vi "UPCONVERSION.vi"() -> ()   [LabVIEW 2011]
uses:
  Control 1.ctl
  Control 2.ctl
  <vilib>/Utility/file.llb/Write To Spreadsheet File (DBL).vi
panel:
  out "error out":errorcluster
  out "No of Scan":i32
  in  "Stop Taking Data":bool
  in  "UP CONVERSION":T1(tab)
  in  "Position (mm)":dbl
  out "Current position (mm)":dbl
  in  "Start Data Accusition":bool
  out "Position Time Zero":dbl
  in  "Path for Transients":T2="C:\\Users\\Labuser\\Desktop\\Upconversion_data\\"
  in  "Path for final Averaged Data":T3=path "C:/Users/Labuser/Desktop/Upconversion_data/final"
  in  "50 fs":i32
  in  "250 fs":i32
  in  "1ps":i32
  in  "5ps":i32
  out "GRAPH":T4(graph)
  out "XY Graph":cluster{"Y":dbl[], "Y":dbl[]}[](graph)
  out "Final Graph":cluster{"Y":dbl[], "Y":dbl[]}[](graph)
  # "50,20.50,40,t0=117.65"
  # "Enter number of steps"
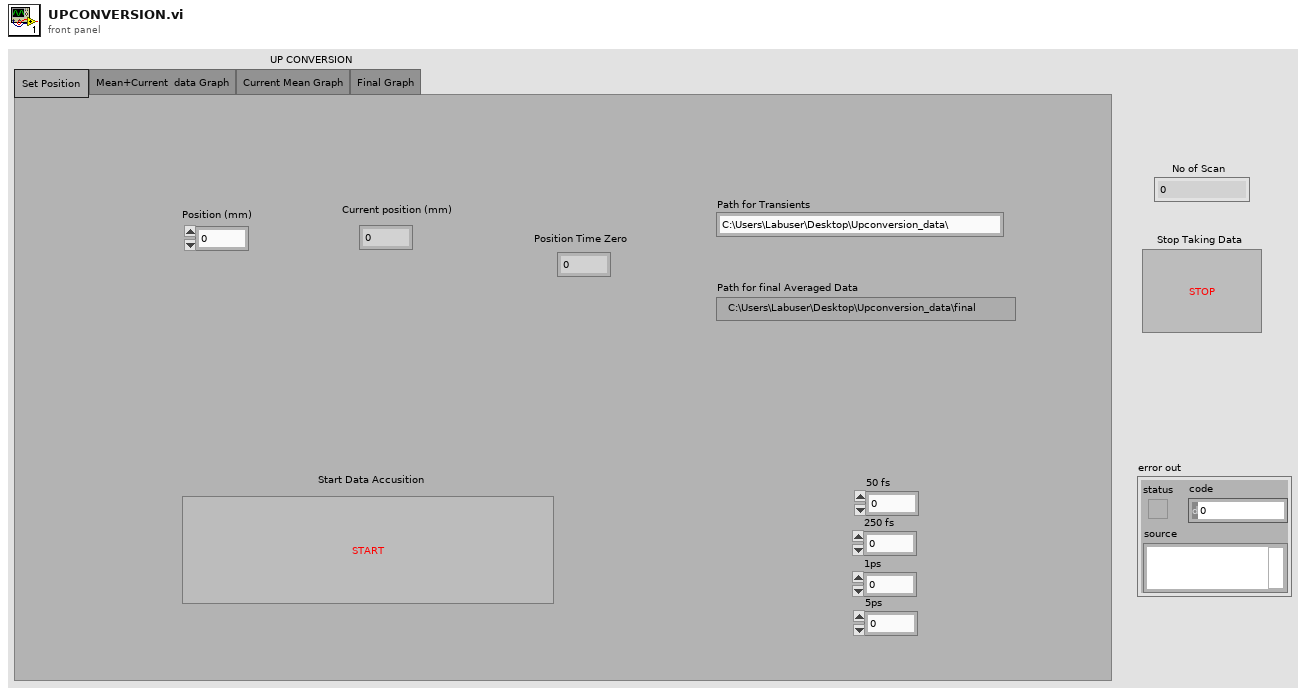
[diagram p1: front panel]
types:
  T1 = enum32{"Set Position ", "Mean+Current  data Graph", "Current Mean Graph", "Final Graph"}
  T2 = typedef "Control 1.ctl" = string
  T3 = typedef "Control 2.ctl" = path
  T4 = cluster{"XY Graph ":cluster{"Y":dbl[], "Y":dbl[]}[], "XY Graph":cluster{"Y":dbl[], "Y":dbl[]}[]}
  T5 = enum16{"open", "replace", "create", "open or create", "replace or create", "replace or create with confirmation"}
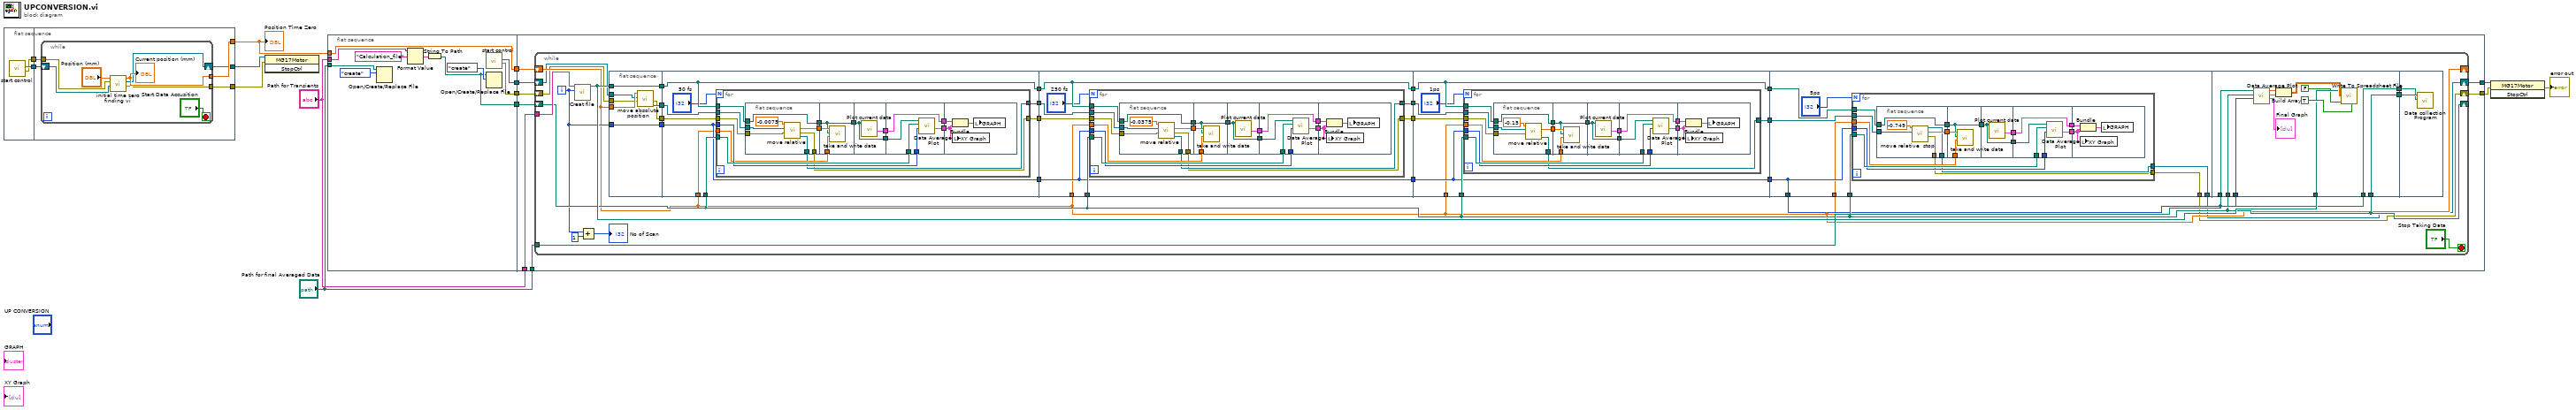
[diagram p0: block diagram]
diagram:
  n1 = flat-sequence {
    tunnel: [w16] -> w2
    tunnel: [w15] -> w1
    tunnel: [w21] -> w14
    tunnel: [w20] -> w9
    tunnel: [w19] -> w6
    tunnel: w2 -> [w18]
    tunnel: w1 -> [w17]
    frame #0 {
      n2 = call "start control.vi"() -> ("error out"=w15:errorcluster, "reference out"=w16:refnum<k7>)  [unwired: 10 in]
    }
    frame #1 {
      n3 = while {
        tunnel: [w26] -> w21
        tunnel: [w25] -> w19
        tunnel: w17 -> [w23]
        shift-right: [w22] -> w20
        shift-left: w18 -> [w24]
        stop <- "Start Data Accusition" stop-if-true
        n4 = call "initial time zero finding vi.vi"("reference"=w24, "error in (no error)"=w23, "absolute displacment"="Position (mm)") -> ("error out"=w25:errorcluster, "reference out"=w22:refnum<k7>, "Current Position"=w26:sgl)  [unwired: 6 in]
        "Current position (mm)" <- w26
      }
    }
  }
  n5 = invoke class="MG17Motor" method="StopCtrl"(reference=w9, error in=w6) -> ()  [unwired: 1 in, 3 out]
  n6 = flat-sequence {
    tunnel: w14 -> [w38]
    tunnel: [w38] -> w13
    tunnel: [w33] -> w12
    tunnel: "Path for final Averaged Data" -> [w37]
    tunnel: "Path for Transients" -> [w32]
    tunnel: [w30] -> w8
    tunnel: [w29] -> w7
    tunnel: "Path for final Averaged Data" -> [w43]
    tunnel: "Path for Transients" -> [w44]
    tunnel: w12 -> [w45]
    tunnel: w13 -> [w46]
    tunnel: w8 -> [w42]
    tunnel: w7 -> [w41]
    tunnel: [w40] -> w5
    tunnel: [w39] -> w4
    frame #0 {
      n7 = Open/Create/Replace File(file path (use dialog)=w37, operation (0:open)=T5."create") -> ()  [unwired: 4 in, 3 out]
      n8 = Format Value(string ("")=w32, format string="Calculation_file") -> (output string=w34:string)  [unwired: 1 in]
      n9 = String To Path(string=w34) -> (path=w33:path)
      n10 = call "start control.vi"() -> ("error out"=w29:errorcluster, "reference out"=w30:refnum<k7>)  [unwired: 10 in]
      n11 = Open/Create/Replace File(file path (use dialog)=w33, operation (0:open)=T5."create") -> ()  [unwired: 4 in, 3 out]
    }
    frame #1 {
      n12 = while {
        shift-right: [w55] -> _
        shift-left: w46 -> [w55]
        shift-right: [w65] -> _
        shift-left: w45 -> [w65]
        tunnel: w44 -> [w68]
        tunnel: w43 -> [w67]
        shift-right: [w48] -> w40
        shift-left: w42 -> [w53]
        shift-right: [w47] -> w39
        shift-left: w41 -> [w52]
        i -> [w63]
        stop <- "Stop Taking Data" stop-if-true
        n13 = call "Creat file.vi"("Numeric"=w63, "File Path"=w68) -> ("Path"=w66:path)  [unwired: 9 in]
        n14 = Add(x=w63, y=1) -> (x+y=→"No of Scan":i32)
        n15 = flat-sequence {
          tunnel: [w84] -> w77
          tunnel: w66 -> [w84]
          tunnel: w63 -> [w83]
          tunnel: [w83] -> w72
          tunnel: w55 -> [w82]
          tunnel: [w81] -> w54
          tunnel: w53 -> [w80]
          tunnel: w52 -> [w79]
          tunnel: [w78] -> w51
          tunnel: w77 -> [w93]
          tunnel: [w93] -> w76
          tunnel: w65 -> [w92]
          tunnel: w72 -> [w91]
          tunnel: [w91] -> w71
          tunnel: w55 -> [w90]
          tunnel: [w88] -> w58
          tunnel: w54 -> [w87]
          tunnel: w51 -> [w86]
          tunnel: [w85] -> w50
          tunnel: w76 -> [w137]
          tunnel: [w137] -> w74
          tunnel: w65 -> [w136]
          tunnel: w71 -> [w135]
          tunnel: [w135] -> w70
          tunnel: w55 -> [w134]
          tunnel: w58 -> [w132]
          tunnel: [w131] -> w57
          tunnel: w50 -> [w130]
          tunnel: [w129] -> w49
          tunnel: [w180] -> w75
          tunnel: w74 -> [w180]
          tunnel: w65 -> [w179]
          tunnel: w70 -> [w178]
          tunnel: [w178] -> w69
          tunnel: w55 -> [w177]
          tunnel: w57 -> [w175]
          tunnel: [w174] -> w56
          tunnel: w49 -> [w173]
          tunnel: w75 -> [w221]
          tunnel: w65 -> [w220]
          tunnel: w69 -> [w219]
          tunnel: [w219] -> w64
          tunnel: w55 -> [w218]
          tunnel: w56 -> [w216]
          tunnel: [w215] -> w48
          tunnel: [w214] -> w47
          tunnel: w67 -> [w261]
          tunnel: w66 -> [w260]
          tunnel: w65 -> [w259]
          tunnel: w64 -> [w258]
          tunnel: w66 -> [w255]
          tunnel: w65 -> [w256]
          tunnel: [w256] -> w60
          tunnel: [w255] -> w59
          tunnel: w60 -> [w268]
          tunnel: w59 -> [w267]
          frame #0 {
            n16 = call "move absolute position.vi"("error in (no error)"=w79, "reference"=w80, "absolute displacment"=w82) -> ("reference out"=w81:refnum<k7>, "error out"=w78:errorcluster)  [unwired: 6 in, 1 out]
          }
          frame #1 {
            n17 = for {
              N: "50 fs" -> [_]
              tunnel: w93 -> [w108]
              tunnel: w92 -> [w104]
              tunnel: w91 -> [w101]
              tunnel: w90 -> [w100]
              tunnel: [w97] -> w88
              tunnel: w87 -> [w96]
              tunnel: w86 -> [w95]
              tunnel: [w94] -> w85
              n18 = flat-sequence {
                tunnel: [w113] -> w99
                tunnel: [w115] -> w98
                tunnel: w108 -> [w115]
                tunnel: [w112] -> w97
                tunnel: w96 -> [w111]
                tunnel: w95 -> [w110]
                tunnel: [w109] -> w94
                tunnel: [w117] -> w107
                tunnel: w100 -> [w116]
                tunnel: w98 -> [w117]
                tunnel: w99 -> [w118]
                tunnel: w107 -> [w119]
                tunnel: [w120] -> w106
                tunnel: [w119] -> w103
                tunnel: w106 -> [w125]
                tunnel: [w125] -> w105
                tunnel: w104 -> [w124]
                tunnel: w103 -> [w123]
                tunnel: [w122] -> w102
                tunnel: w101 -> [w121]
                tunnel: w105 -> [w127]
                tunnel: w102 -> [w126]
                frame #0 {
                  n19 = call "move relative.vi"("error in (no error)"=w110, "reference"=w111, "relative displacment"=-0.0075 ("Step Size 1")) -> ("reference out"=w112:refnum<k7>, "error out"=w109:errorcluster, "Current Position"=w113:sgl)  [unwired: 6 in]
                }
                frame #1 {
                  n20 = call "take and write data.vi"("y"=w116, "Path"=w117, "Current position (units)"=w118) -> ()  [unwired: 9 in]
                }
                frame #2 {
                  n21 = call "Plot current data.vi"("file path (dialog if empty)"=w119) -> ("XY Graph"=w120:cluster{"Y":dbl[], "Y":dbl[]}[])  [unwired: 8 in]
                }
                frame #3 {
                  n22 = call "Data Average Plot.vi"("No of element"=w121, "Average file path"=w124, "Current file path"=w123) -> ("XY Graph"=w122:cluster{"Y":dbl[], "Y":dbl[]}[])  [unwired: 4 in, 2 out]
                }
                frame #4 {
                  n23 = Bundle("XY Graph"=w127, "XY Graph"=w126) -> (w128:T4)  [unwired: 1 in]
                  n24 = local write "XY Graph"(w126) -> ()
                  n25 = local write "GRAPH"(w128) -> ()
                }
              }
            }
          }
          frame #2 {
            n26 = for {
              N: "250 fs" -> [_]
              tunnel: w137 -> [w152]
              tunnel: w136 -> [w148]
              tunnel: w135 -> [w145]
              tunnel: w134 -> [w144]
              tunnel: w132 -> [w141]
              tunnel: [w140] -> w131
              tunnel: w130 -> [w139]
              tunnel: [w138] -> w129
              n27 = flat-sequence {
                tunnel: [w157] -> w143
                tunnel: [w159] -> w142
                tunnel: w152 -> [w159]
                tunnel: w141 -> [w156]
                tunnel: [w155] -> w140
                tunnel: w139 -> [w154]
                tunnel: [w153] -> w138
                tunnel: [w161] -> w151
                tunnel: w144 -> [w160]
                tunnel: w142 -> [w161]
                tunnel: w143 -> [w162]
                tunnel: w151 -> [w163]
                tunnel: [w164] -> w150
                tunnel: [w163] -> w147
                tunnel: w150 -> [w169]
                tunnel: [w169] -> w149
                tunnel: w148 -> [w168]
                tunnel: w147 -> [w167]
                tunnel: [w166] -> w146
                tunnel: w145 -> [w165]
                tunnel: w149 -> [w171]
                tunnel: w146 -> [w170]
                frame #0 {
                  n28 = call "move relative.vi"("error in (no error)"=w154, "reference"=w156, "relative displacment"=-0.0375 ("Step Size 2")) -> ("reference out"=w155:refnum<k7>, "error out"=w153:errorcluster, "Current Position"=w157:sgl)  [unwired: 6 in]
                }
                frame #1 {
                  n29 = call "take and write data.vi"("y"=w160, "Path"=w161, "Current position (units)"=w162) -> ()  [unwired: 9 in]
                }
                frame #2 {
                  n30 = call "Plot current data.vi"("file path (dialog if empty)"=w163) -> ("XY Graph"=w164:cluster{"Y":dbl[], "Y":dbl[]}[])  [unwired: 8 in]
                }
                frame #3 {
                  n31 = call "Data Average Plot.vi"("No of element"=w165, "Average file path"=w168, "Current file path"=w167) -> ("XY Graph"=w166:cluster{"Y":dbl[], "Y":dbl[]}[])  [unwired: 4 in, 2 out]
                }
                frame #4 {
                  n32 = Bundle("XY Graph"=w171, "XY Graph"=w170) -> (w172:T4)  [unwired: 1 in]
                  n33 = local write "XY Graph"(w170) -> ()
                  n34 = local write "GRAPH"(w172) -> ()
                }
              }
            }
          }
          frame #3 {
            n35 = for {
              N: "1ps" -> [_]
              tunnel: w180 -> [w194]
              tunnel: w179 -> [w190]
              tunnel: w178 -> [w187]
              tunnel: w177 -> [w186]
              tunnel: w175 -> [w183]
              tunnel: [w182] -> w174
              tunnel: w173 -> [w181]
              n36 = flat-sequence {
                tunnel: [w197] -> w185
                tunnel: [w200] -> w184
                tunnel: w194 -> [w200]
                tunnel: w183 -> [w199]
                tunnel: [w196] -> w182
                tunnel: w181 -> [w195]
                tunnel: [w202] -> w193
                tunnel: w186 -> [w201]
                tunnel: w184 -> [w202]
                tunnel: w185 -> [w203]
                tunnel: w193 -> [w204]
                tunnel: [w205] -> w192
                tunnel: [w204] -> w189
                tunnel: w192 -> [w210]
                tunnel: [w210] -> w191
                tunnel: w190 -> [w209]
                tunnel: w189 -> [w208]
                tunnel: [w207] -> w188
                tunnel: w187 -> [w206]
                tunnel: w191 -> [w212]
                tunnel: w188 -> [w211]
                frame #0 {
                  n37 = call "move relative.vi"("error in (no error)"=w195, "reference"=w199, "relative displacment"=-0.15 ("Step Size 3")) -> ("reference out"=w196:refnum<k7>, "Current Position"=w197:sgl)  [unwired: 6 in, 1 out]
                }
                frame #1 {
                  n38 = call "take and write data.vi"("y"=w201, "Path"=w202, "Current position (units)"=w203) -> ()  [unwired: 9 in]
                }
                frame #2 {
                  n39 = call "Plot current data.vi"("file path (dialog if empty)"=w204) -> ("XY Graph"=w205:cluster{"Y":dbl[], "Y":dbl[]}[])  [unwired: 8 in]
                }
                frame #3 {
                  n40 = call "Data Average Plot.vi"("No of element"=w206, "Average file path"=w209, "Current file path"=w208) -> ("XY Graph"=w207:cluster{"Y":dbl[], "Y":dbl[]}[])  [unwired: 4 in, 2 out]
                }
                frame #4 {
                  n41 = Bundle("XY Graph"=w212, "XY Graph"=w211) -> (w213:T4)  [unwired: 1 in]
                  n42 = local write "XY Graph"(w211) -> ()
                  n43 = local write "GRAPH"(w213) -> ()
                }
              }
            }
          }
          frame #4 {
            n44 = for {
              N: "5ps" -> [_]
              tunnel: w221 -> [w235]
              tunnel: w220 -> [w231]
              tunnel: w219 -> [w228]
              tunnel: w218 -> [w227]
              tunnel: w216 -> [w224]
              tunnel: [w223] -> w215
              tunnel: [w222] -> w214
              n45 = flat-sequence {
                tunnel: [w238] -> w226
                tunnel: [w241] -> w225
                tunnel: w235 -> [w241]
                tunnel: w224 -> [w239]
                tunnel: [w237] -> w223
                tunnel: [w236] -> w222
                tunnel: [w243] -> w234
                tunnel: w227 -> [w242]
                tunnel: w225 -> [w243]
                tunnel: w226 -> [w244]
                tunnel: w234 -> [w245]
                tunnel: [w246] -> w233
                tunnel: [w245] -> w230
                tunnel: w233 -> [w251]
                tunnel: [w251] -> w232
                tunnel: w231 -> [w250]
                tunnel: w230 -> [w249]
                tunnel: [w248] -> w229
                tunnel: w228 -> [w247]
                tunnel: w232 -> [w253]
                tunnel: w229 -> [w252]
                frame #0 {
                  n46 = call "move relative  stop.vi"("reference"=w239, "relative displacment"=-0.749 ("Step Size 4")) -> ("error out"=w236:errorcluster, "Current Position"=w238:sgl, "reference out"=w237:refnum<k7>)  [unwired: 7 in]
                }
                frame #1 {
                  n47 = call "take and write data.vi"("y"=w242, "Path"=w243, "Current position (units)"=w244) -> ()  [unwired: 9 in]
                }
                frame #2 {
                  n48 = call "Plot current data.vi"("file path (dialog if empty)"=w245) -> ("XY Graph"=w246:cluster{"Y":dbl[], "Y":dbl[]}[])  [unwired: 8 in]
                }
                frame #3 {
                  n49 = call "Data Average Plot.vi"("No of element"=w247, "Average file path"=w250, "Current file path"=w249) -> ("XY Graph"=w248:cluster{"Y":dbl[], "Y":dbl[]}[])  [unwired: 4 in, 2 out]
                }
                frame #4 {
                  n50 = Bundle("XY Graph"=w253, "XY Graph"=w252) -> (w254:T4)  [unwired: 1 in]
                  n51 = local write "XY Graph"(w252) -> ()
                  n52 = local write "GRAPH"(w254) -> ()
                }
              }
            }
          }
          frame #5 {
            n53 = call "Data Average Plot.vi"("No of element"=w258, "Average file path"=w259, "Current file path"=w260) -> ("XY Graph"=→"Final Graph":cluster{"Y":dbl[], "Y":dbl[]}[], "Y Out"=w264:dbl[], "X Out"=w263:dbl[])  [unwired: 4 in]
            n54 = Build Array(w263, w264) -> (w265:dbl[][])
            n55 = call-poly <vilib>:"Write To Spreadsheet File.vi"("transpose? (no:F)"=TRUE, "append to file? (new file:F)"=FALSE, "2D data"=w265, "file path (dialog if empty)"=w261) -> ()  [unwired: 4 in, 1 out]
          }
          frame #6 {
            n56 = call "Data collection Program.vi"("Current File Name"=w267, "Average file path"=w268) -> ()  [unwired: 9 in, 1 out]
          }
        }
      }
    }
  }
  n57 = invoke class="MG17Motor" method="StopCtrl"(reference=w5, error in=w4) -> (error out=→"error out":errorcluster)  [unwired: 1 in, 2 out]
  "Position Time Zero" <- w14
